vi "LoadController.vi"(8 "error in (no error)":errorcluster, 10 "Actor In":refnum<class "Actor.lvclass">, 11 "Microscope_RM21 in":refnum<class "Microscope_RM21.lvclass">) -> (0 "error out":errorcluster, 3 "Microscope_RM21 out":refnum<class "Microscope_RM21.lvclass">)   [LabVIEW 2020, in "Microscope_RM21.lvlib" / "Microscope_RM21.lvclass"]
uses:
  Microscope_RM21.lvclass
  <vilib>/ActorFramework/Actor/Actor.lvclass
  ViewController/Microscope Controller/Microscope Controller.lvclass
  C:/Program Files/National Instruments/LabVIEW 2020/vi.lib/ActorFramework/Actor/Actor.lvclass
  Hardware Abstraction Layer/Microscope/Microscope/Microscope.lvclass
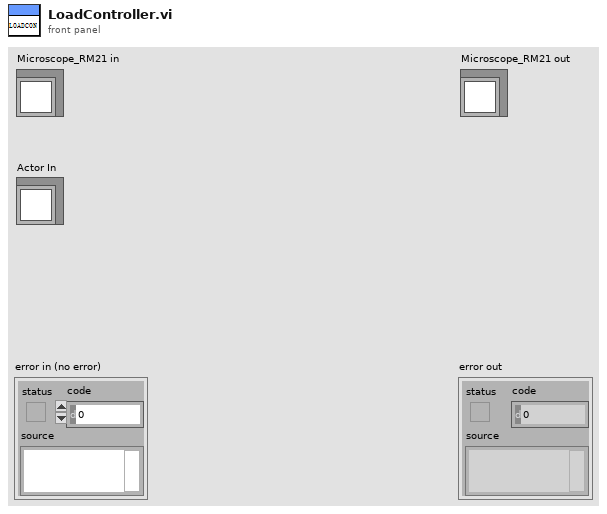
[diagram p1: front panel]
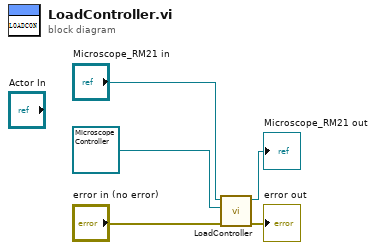
[diagram p0: block diagram]
diagram:
  n1 = call-parent "LoadController.vi"("error in (no error)"="error in (no error)", "Actor In"=refnum<class "Microscope Controller.lvclass"> refnum ("Microscope Controller.lvlib:Microscope Controller.lvclass"), "Microscope in"="Microscope_RM21 in") -> ("error out"=→"error out":errorcluster, "Microscope out"=→"Microscope_RM21 out":refnum<class "Microscope_RM21.lvclass">)  [unwired: 7 in]
